vi "Bemerkung.vi"(5 "Table Configuration":T1={"Table Settings"={"Number of Columns"=1, "Width (%)"=100.0, "Relative Column Widths (%)"=[100.0], "Horizontal Align"=0, "Header Rows"=0}, "Cell Defaults"={"Background Color"=16777215, "Horizontal Align"=3, "Vertical Align"=1, "Minimum Height"=0.0, "Fixed Height"=0.0, "Padding"={"Left"=2.0, "Top"=2.0, "Right"=2.0, "Bottom"=3.0}}, "Borders"={"Left"={"Enabled"=FALSE, "Width"=1.0, "Color"=16777215}, "Top"={"Enabled"=FALSE, "Width"=1.0, "Color"=16777215}, "Right"={"Enabled"=FALSE, "Width"=1.0, "Color"=16777215}, "Bottom"={"Enabled"=FALSE, "Width"=1.0, "Color"=16777215}, "Middle Horizontal"={"Enabled"=FALSE, "Width"=0.5, "Color"=16777215}, "Middle Vertical"={"Enabled"=FALSE, "Width"=0.5, "Color"=16777215}}} {"Cell Defaults"."Vertical Align" items=["Bottom", "Middle", "Top"]; "Cell Defaults"."Horizontal Align" items=["Center", "Justified", "JustifiedAll", "Left", "Right"]; "Table Settings"."Horizontal Align" items=["Center"=0, "Left"=3, "Right"=4]}, 7 "Cell Configuration":T5={"Cell Defaults"={"Background Color"=16777215, "Horizontal Align"=3, "Vertical Align"=1, "Minimum Height"=0.0, "Fixed Height"=0.0, "Padding"={"Left"=2.0, "Top"=2.0, "Right"=2.0, "Bottom"=3.0}}, "Borders"={"Left"={"Enabled"=FALSE, "Width"=1.0, "Color"=0}, "Top"={"Enabled"=FALSE, "Width"=1.0, "Color"=0}, "Right"={"Enabled"=FALSE, "Width"=1.0, "Color"=0}, "Bottom"={"Enabled"=FALSE, "Width"=1.0, "Color"=0}}, "Column Span"=0} {"Cell Defaults"."Vertical Align" items=["Bottom", "Middle", "Top"]; "Cell Defaults"."Horizontal Align" items=["Center", "Justified", "JustifiedAll", "Left", "Right"]}, 8 "Fehler (Eingang, kein Fehler)":errorcluster, 9 "Index":i32, 10 "Bemerkung":T6[](array[typedef]) {"Align (Left)" items=["Center", "Justified", "Justified All", "Left", "Right"]}, 11 "Context (Eingang)":refnum<class "Context.lvclass">) -> (0 "Fehler (Ausgang)":errorcluster, 3 "Context (Ausgang)":refnum<class "Context.lvclass">)   [LabVIEW 2020, in "PDF Interface.lvlib" / "PDF Interface Helper.lvlib"]
uses:
  PDF Interface Helper.lvlib
  PDFBemerkung.ctl
  <vilib>/Simplicity AI/SAI_PDF_API/Classes/Context/Controls/SAI_PDF_Text Align.ctl
  <vilib>/Simplicity AI/SAI_PDF_API/Classes/Context/Controls/SAI_PDF_Font.ctl
  <vilib>/Simplicity AI/SAI_PDF_API/Classes/Context/Controls/SAI_PDF_Font Encoding.ctl
  <vilib>/Simplicity AI/SAI_PDF_API/Classes/Context/Context.lvclass
  <vilib>/Simplicity AI/SAI_PDF_API/Classes/Table Builder/Controls/SAI_PDF_Cell Configuration.ctl
  <vilib>/Simplicity AI/SAI_PDF_API/Classes/Table Builder/Controls/SAI_PDF_Default Cell Format.ctl
  <vilib>/Simplicity AI/SAI_PDF_API/Classes/Table Builder/Controls/SAI_PDF_BorderLine.ctl
  <vilib>/Simplicity AI/SAI_PDF_API/Classes/Table Builder/Controls/SAI_PDF_Table Configuration.ctl
  <vilib>/Simplicity AI/SAI_PDF_API/Classes/Table Builder/Controls/SAI_PDF_Table Horizontal Align.ctl
  <vilib>/Simplicity AI/SAI_PDF_API/Classes/Context/Methods/Public/Low Level/Add/SAI_PDF_Add Line Feed.vi
  <vilib>/Simplicity AI/SAI_PDF_API/Classes/Context/Methods/Public/Low Level/Add/SAI_PDF_Add Paragraph.vi
  <vilib>/Simplicity AI/SAI_PDF_API/Classes/Table Builder/Table Builder.lvclass
panel:
  # "(Cp1252)"
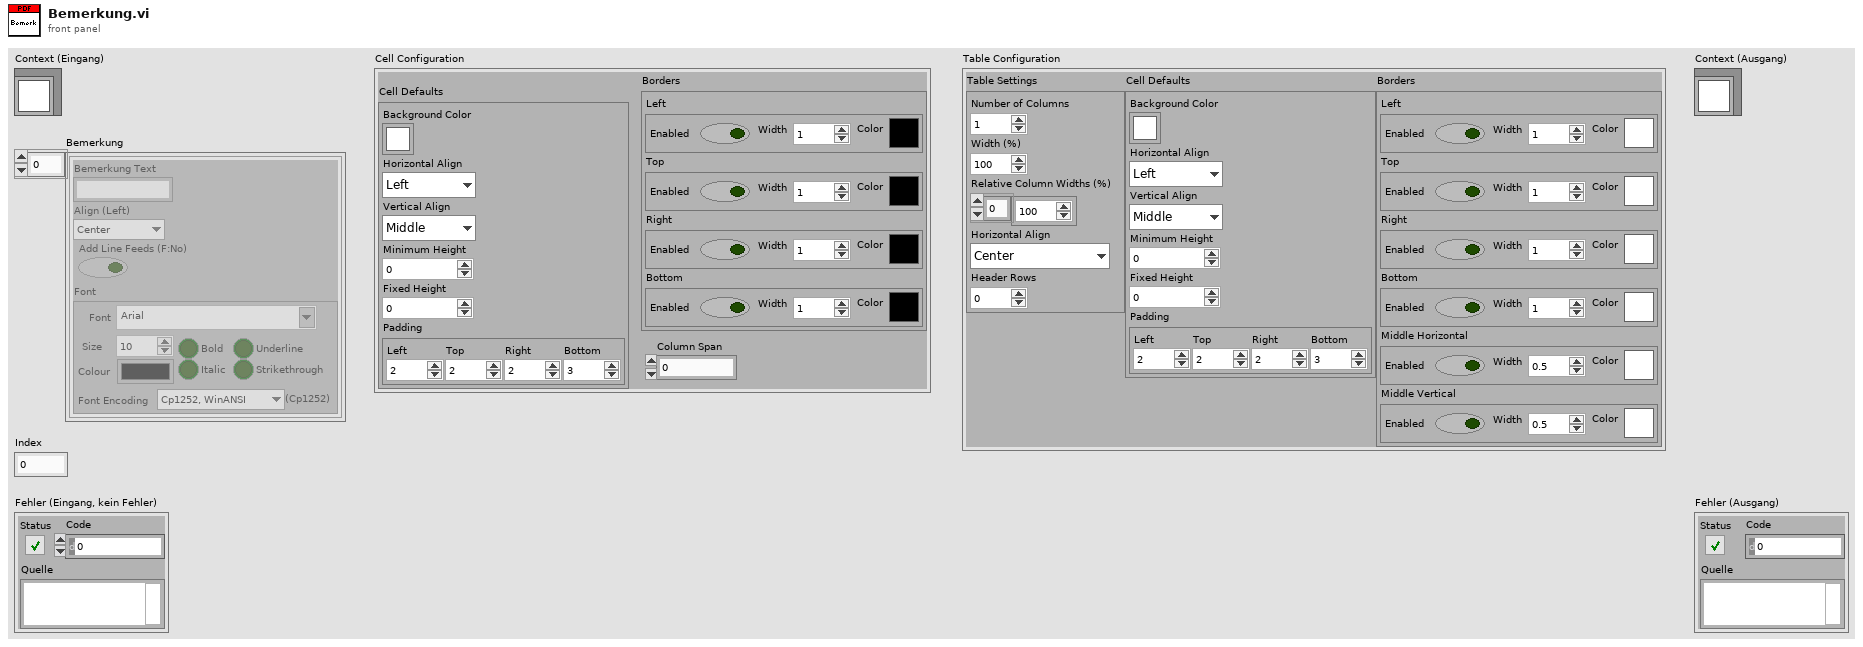
[diagram p1: front panel]
types:
  T1 = typedef "SAI_PDF_Toolkit.lvlib/Table Builder.lvclass/SAI_PDF_Table Configuration.ctl" = cluster{"Table Settings":cluster{"Number of Columns":i32, "Width (%)":sgl, "Relative Column Widths (%)":sgl[], "Horizontal Align":T2, "Header Rows":i32}, "Cell Defaults":T3, "Borders":cluster{"Left":T4, "Top":T4, "Right":T4, "Bottom":T4, "Middle Horizontal":T4, "Middle Vertical":T4}}
  T2 = typedef "SAI_PDF_Toolkit.lvlib/Table Builder.lvclass/SAI_PDF_Table Horizontal Align.ctl" = i32
  T3 = typedef "SAI_PDF_Toolkit.lvlib/Table Builder.lvclass/SAI_PDF_Default Cell Format.ctl" = cluster{"Background Color":u32, "Horizontal Align":i32, "Vertical Align":i32, "Minimum Height":sgl, "Fixed Height":sgl, "Padding":cluster{"Left":sgl, "Top":sgl, "Right":sgl, "Bottom":sgl}}
  T4 = typedef "SAI_PDF_Toolkit.lvlib/Table Builder.lvclass/SAI_PDF_BorderLine.ctl" = cluster{"Enabled":bool, "Width":sgl, "Color":u32}
  T5 = typedef "SAI_PDF_Toolkit.lvlib/Table Builder.lvclass/SAI_PDF_Cell Configuration.ctl" = cluster{"Cell Defaults":T3, "Borders":cluster{"Left":T4, "Top":T4, "Right":T4, "Bottom":T4}, "Column Span":i32}
  T6 = typedef "PDF Interface.lvlib/PDF Interface Helper.lvlib/PDFBemerkung.ctl" = cluster{"Bemerkung Text":string, "Align (Left)":T7, "Add Line Feeds (F:No)":bool, "Font":T8}
  T7 = typedef "SAI_PDF_Toolkit.lvlib/Context.lvclass/SAI_PDF_Text Align.ctl" = i32
  T8 = typedef "SAI_PDF_Toolkit.lvlib/Context.lvclass/SAI_PDF_Font.ctl" = cluster{"Font":string, "Size":i32, "Colour":u32, "Bold":bool, "Italic":bool, "Underline":bool, "Strikethrough":bool, "Font Encoding":T9}
  T9 = typedef "SAI_PDF_Toolkit.lvlib/Context.lvclass/SAI_PDF_Font Encoding.ctl" = enum16{"Cp1252, WinANSI", "IdentityH", "IdentityV", "Cp1250", "Cp1257", "MacRoman"}
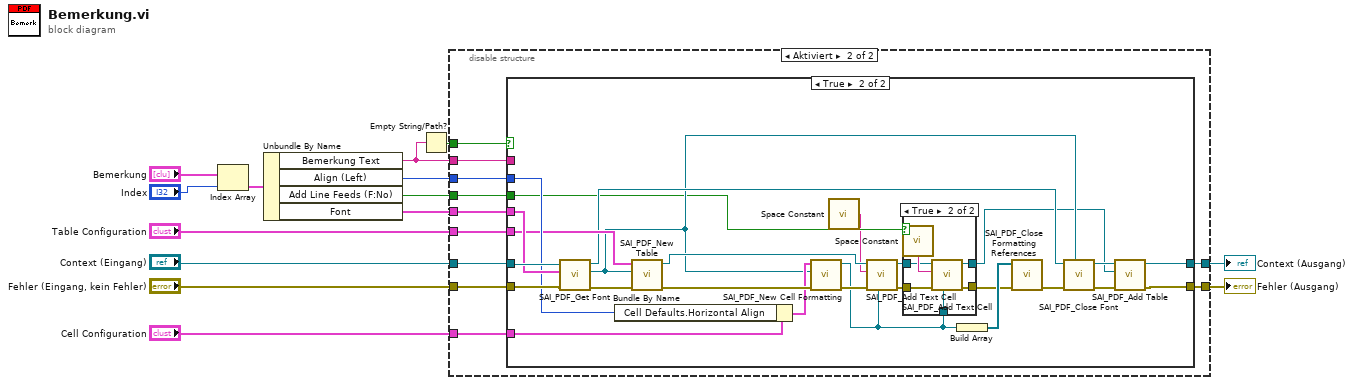
[diagram p0: block diagram]
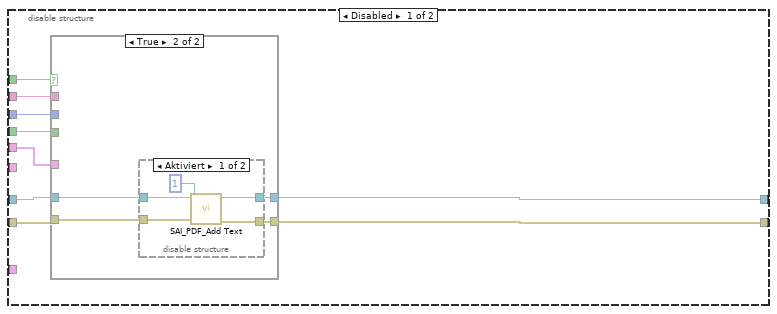
[diagram p2: hidden frame]
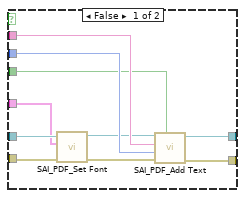
[diagram p3: hidden frame]
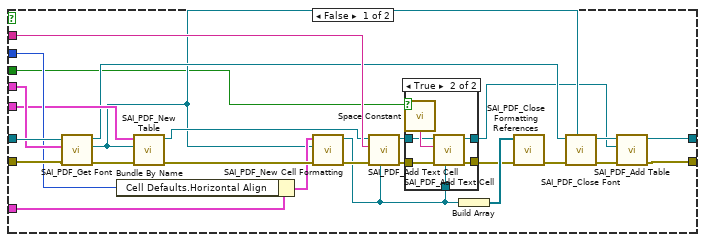
[diagram p5: hidden frame]
diagram:
  n1 = Index Array(array="Bemerkung", index="Index") -> (element=w9:T6)
  n2 = Unbundle By Name(w9) -> ("Bemerkung Text"=w11:string, "Align (Left)"=w12:T7, "Add Line Feeds (F:No)"=w13:bool, "Font"=w1:T8)
  n3 = Empty String/Path?(string/path=w11) -> (empty?=w10:bool)
  n4 = disable-structure shown="Aktiviert" {
    disable-tunnel: w13 -> [w23 w45]
    disable-tunnel: w12 -> [w22 w51]
    disable-tunnel: w11 -> [w21 w48]
    disable-tunnel: w10 -> [w20 w55]
    disable-tunnel: "Fehler (Eingang, kein Fehler)" -> [w19 w52]
    disable-tunnel: [w18 w47] -> w6
    disable-tunnel: [w17 w46] -> w5
    disable-tunnel: "Context (Eingang)" -> [w16 w54]
    disable-tunnel: w1 -> [w15 w53]
    disable-tunnel: "Cell Configuration" -> [_ w50]
    disable-tunnel: "Table Configuration" -> [_ w49]
    frame Disabled {
      n5 = case shown="True" w20 {
        tunnel: w16 -> [w28 w37]
        tunnel: [w33 w36] -> w17
        tunnel: [w32 w34] -> w18
        tunnel: w19 -> [w26 w35]
        tunnel: w21 -> [w31 _]
        tunnel: w22 -> [w30 _]
        tunnel: w23 -> [w29 _]
        tunnel: w15 -> [w24 _]
        frame False {
          n6 = call <vilib>:"SAI_PDF_Set Font.vi"("error in"=w26, "Font"=w24, "Context In"=w28) -> ("error out"=w25:errorcluster, "Context Out"=w27:refnum<class "Context.lvclass">)  [unwired: 7 out]
          n7 = call-poly <vilib>:"SAI_PDF_Add Text.vi"("Add Line Feeds (F:No)"=w29, "error in"=w25, "Align (Left)"=w30, "Text"=w31, "Context In"=w27) -> ("error out"=w32:errorcluster, "Context Out"=w33:refnum<class "Context.lvclass">)  [unwired: 5 out]
        }
        frame True {
          n8 = disable-structure shown="Aktiviert" {
            disable-tunnel: w37 -> [w42 w44]
            disable-tunnel: [w41 w44] -> w36
            disable-tunnel: w35 -> [w40 w43]
            disable-tunnel: [w39 w43] -> w34
            frame Enabled {
              n9 = call-poly <vilib>:"SAI_PDF_Add Text.vi"("error in"=w40, "Number of Lines (1)"=u32 1, "Context In"=w42) -> ("error out"=w39:errorcluster, "Context Out"=w41:refnum<class "Context.lvclass">)  [unwired: 7 out]
            }
            frame Disabled {
            }
          }
        }
      }
    }
    frame Enabled {
      n10 = case shown="True" w55 {
        tunnel: w54 -> [w81 w115]
        tunnel: w53 -> [w80 w114]
        tunnel: w52 -> [w79 w113]
        tunnel: w51 -> [w76 w110]
        tunnel: w50 -> [w74 w108]
        tunnel: w49 -> [w73 w107]
        tunnel: w48 -> [w71 _]
        tunnel: [w63 w98] -> w47
        tunnel: [w62 w97] -> w46
        tunnel: w45 -> [w56 w91]
        frame False {
          n11 = call <vilib>:"SAI_PDF_Get Font.vi"("error in"=w79, "Font"=w80, "Context In"=w81) -> ("error out"=w77:errorcluster, "Font"=w66:refnum<class "Font.lvclass">, "Context Out"=w67:refnum<class "Context.lvclass">)  [unwired: 6 out]
          n12 = Bundle By Name(cluster=w74, "Cell Defaults.Horizontal Align"=w76) -> (w75:T5)
          n13 = call <vilib>:"SAI_PDF_New Table.vi"("error in"=w77, "Font In"=w66, "Table Configuration"=w73) -> ("error out"=w78:errorcluster, "Table Builder"=w70:refnum<class "Table Builder.lvclass">)  [unwired: 7 out]
          n14 = call <vilib>:"SAI_PDF_New Cell Formatting.vi"("error in"=w78, "Font In"=w66, "Cell Configuration"=w75) -> ("error out"=w72:errorcluster, "Cell Formatting"=w57:refnum<class "Formatting.lvclass">)  [unwired: 7 out]
          n15 = call <vilib>:"SAI_PDF_Add Text Cell.vi"("Formatting In"=w57, "error in"=w72, "Text"=w71, "Table Builder In"=w70) -> ("error out"=w61:errorcluster, "Table Builder Out"=w59:refnum<class "Table Builder.lvclass">)  [unwired: 6 in]
          n16 = case shown="True" w56 {
            tunnel: w61 -> [w82 w89]
            tunnel: [w82 w88] -> w60
            tunnel: w59 -> [w83 w86]
            tunnel: [w83 w85] -> w58
            tunnel: w57 -> [_ w84]
            frame False {
            }
            frame True {
              n17 = call <vilib>:"Space Constant.vi"() -> ("String"=w87:string)
              n18 = call <vilib>:"SAI_PDF_Add Text Cell.vi"("Formatting In"=w84, "error in"=w89, "Text"=w87, "Table Builder In"=w86) -> ("error out"=w88:errorcluster, "Table Builder Out"=w85:refnum<class "Table Builder.lvclass">)  [unwired: 6 in]
            }
          }
          n19 = Build Array(w57) -> (w69:refnum<class "Formatting.lvclass">[])
          n20 = call <vilib>:"SAI_PDF_Close Formatting References.vi"("error in"=w60, "Formatting Refs"=w69) -> ("error out"=w68:errorcluster)  [unwired: 9 out]
          n21 = call <vilib>:"SAI_PDF_Close Font.vi"("Font"=w66, "error in"=w68, "Context In"=w67) -> ("error out"=w64:errorcluster, "Context Out"=w65:refnum<class "Context.lvclass">)  [unwired: 7 out]
          n22 = call <vilib>:"SAI_PDF_Add Table.vi"("error in"=w64, "Table Builder In"=w58, "Context In"=w65) -> ("error out"=w63:errorcluster, "Context Out"=w62:refnum<class "Context.lvclass">)  [unwired: 7 out]
        }
        frame True {
          n23 = call <vilib>:"SAI_PDF_Get Font.vi"("error in"=w113, "Font"=w114, "Context In"=w115) -> ("error out"=w111:errorcluster, "Font"=w101:refnum<class "Font.lvclass">, "Context Out"=w102:refnum<class "Context.lvclass">)  [unwired: 6 out]
          n24 = Bundle By Name(cluster=w108, "Cell Defaults.Horizontal Align"=w110) -> (w109:T5)
          n25 = call <vilib>:"SAI_PDF_New Table.vi"("error in"=w111, "Font In"=w101, "Table Configuration"=w107) -> ("error out"=w112:errorcluster, "Table Builder"=w105:refnum<class "Table Builder.lvclass">)  [unwired: 7 out]
          n26 = call <vilib>:"SAI_PDF_New Cell Formatting.vi"("error in"=w112, "Font In"=w101, "Cell Configuration"=w109) -> ("error out"=w106:errorcluster, "Cell Formatting"=w92:refnum<class "Formatting.lvclass">)  [unwired: 7 out]
          n27 = call <vilib>:"Space Constant.vi"() -> ("String"=w90:string)
          n28 = call <vilib>:"SAI_PDF_Add Text Cell.vi"("Formatting In"=w92, "error in"=w106, "Text"=w90, "Table Builder In"=w105) -> ("error out"=w96:errorcluster, "Table Builder Out"=w94:refnum<class "Table Builder.lvclass">)  [unwired: 6 in]
          n29 = case shown="True" w91 {
            tunnel: w96 -> [w116 w123]
            tunnel: [w116 w122] -> w95
            tunnel: w94 -> [w117 w120]
            tunnel: [w117 w119] -> w93
            tunnel: w92 -> [_ w118]
            frame False {
            }
            frame True {
              n30 = call <vilib>:"Space Constant.vi"() -> ("String"=w121:string)
              n31 = call <vilib>:"SAI_PDF_Add Text Cell.vi"("Formatting In"=w118, "error in"=w123, "Text"=w121, "Table Builder In"=w120) -> ("error out"=w122:errorcluster, "Table Builder Out"=w119:refnum<class "Table Builder.lvclass">)  [unwired: 6 in]
            }
          }
          n32 = Build Array(w92) -> (w104:refnum<class "Formatting.lvclass">[])
          n33 = call <vilib>:"SAI_PDF_Close Formatting References.vi"("error in"=w95, "Formatting Refs"=w104) -> ("error out"=w103:errorcluster)  [unwired: 9 out]
          n34 = call <vilib>:"SAI_PDF_Close Font.vi"("Font"=w101, "error in"=w103, "Context In"=w102) -> ("error out"=w99:errorcluster, "Context Out"=w100:refnum<class "Context.lvclass">)  [unwired: 7 out]
          n35 = call <vilib>:"SAI_PDF_Add Table.vi"("error in"=w99, "Table Builder In"=w93, "Context In"=w100) -> ("error out"=w98:errorcluster, "Context Out"=w97:refnum<class "Context.lvclass">)  [unwired: 7 out]
        }
      }
    }
  }
  "Fehler (Ausgang)" <- w6
  "Context (Ausgang)" <- w5
